vi "GeneratePadLookup.vi"(8 "error in (no error)":errorcluster, 11 "PadLookupRef":refnum<vi>) -> (0 "error out":errorcluster)   [LabVIEW 2012]
uses:
  Controls/PadLookup.ctl
  Controls/PadLookupItem.ctl
  Controls/PadArea.ctl
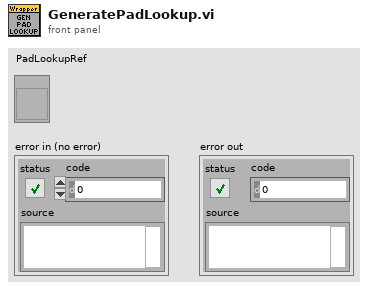
[diagram p1: front panel]
types:
  T1 = typedef "PadLookup.ctl" = cluster{"A":T2, "B":T2, "C":T2, "D":T2, "L":T2, "R":T2, "T":T2, "G":T2}
  T2 = typedef "PadLookupItem.ctl" = cluster{"PadArea":T3, string[]}
  T3 = typedef "PadArea.ctl" = enum16{"CenterA", "CenterB", "CenterC", "CenterD", "L", "R", "T", "G"}
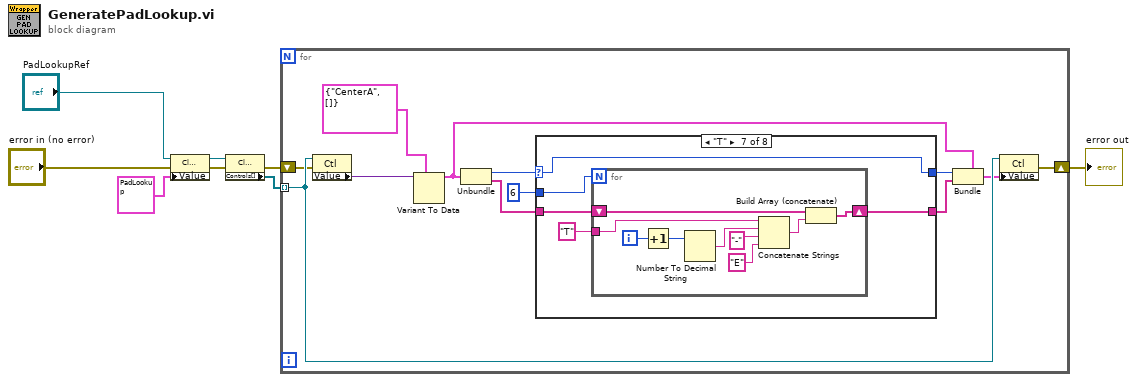
[diagram p0: block diagram]
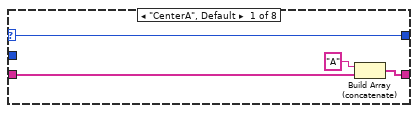
[diagram p2: hidden frame]
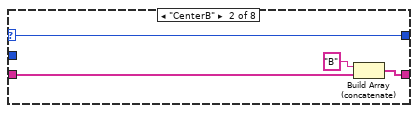
[diagram p3: hidden frame]
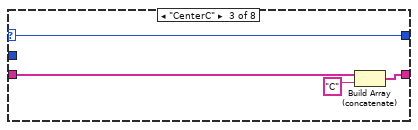
[diagram p4: hidden frame]
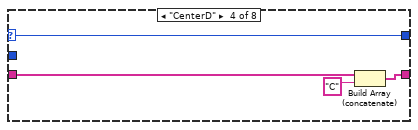
[diagram p5: hidden frame]
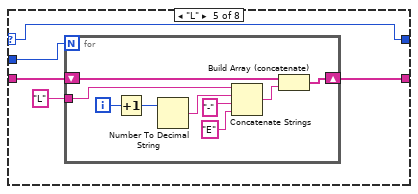
[diagram p6: hidden frame]
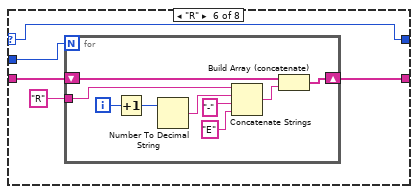
[diagram p7: hidden frame]
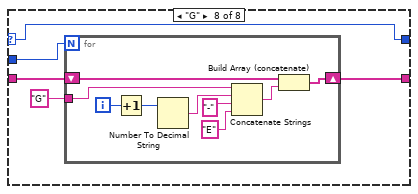
[diagram p8: hidden frame]
diagram:
  n1 = property class="Clust (strict)"(reference="PadLookupRef", error in="error in (no error)", "Value"=T1 {"A"={"PadArea"=enum."CenterA", []}, "B"={"PadArea"=enum."CenterB", []}, "C"={"PadArea"=enum."CenterC", []}, "D"={"PadArea"=enum."CenterD", []}, "L"={"PadArea"=enum."L", []}, "R"={"PadArea"=enum."R", []}, "T"={"PadArea"=enum."T", []}, "G"={"PadArea"=enum."G", []}} ("PadLookup")) -> (reference out=w4:refnum<vi>, error out=w5:errorcluster)
  n2 = property class="Clust (strict)"(reference=w4, error in=w5) -> (error out=w7:errorcluster, "Controls[]"=w3:refnum<vi>[])  [unwired: 1 out]
  n3 = for {
    tunnel: w3 -> [w15] mode=indexing
    shift-right: [w9] -> w8
    shift-left: w7 -> [w10]
    n4 = property class="Ctl"(reference=w15, error in=w10) -> ("Value"=w18:variant)  [unwired: 2 out]
    n5 = Variant To Data(type=T2 {"PadArea"=enum."CenterA", []} ("G"), Variant=w18) -> (data=w16:T2)  [unwired: 1 in, 1 out]
    n6 = Unbundle(w16) -> ("PadArea"=w12:T3, w20:string[])
    n7 = case shown="\"T\"" w12 {
      selector: w12 -> [w22 w26 w31 w34 w39 w53 w67 w81]
      tunnel: w20 -> [w24 w27 w32 w35 w41 w54 w68 w82]
      tunnel: [w22 w26 w31 w34 w39 w53 w67 w81] -> w19
      tunnel: [w21 w25 w29 w33 w40 w52 w66 w80] -> w13
      tunnel: 6 -> [_ _ _ _ w37 w51 w65 w79]
      frame "CenterA", Default {
        n8 = Build Array (concatenate)("A", w24) -> (w21:string[])
      }
      frame "CenterB" {
        n9 = Build Array (concatenate)("B", w27) -> (w25:string[])
      }
      frame "CenterC" {
        n10 = Build Array (concatenate)(w32, "C") -> (w29:string[])
      }
      frame "CenterD" {
        n11 = Build Array (concatenate)(w35, "C") -> (w33:string[])
      }
      frame "L" {
        n12 = for {
          N: w37 -> [_]
          shift-right: [w45] -> w40
          shift-left: w41 -> [w50]
          tunnel: "L" ("string") -> [w44]
          i -> [w49]
          n13 = Increment(x=w49) -> (x+1=w48:i32)
          n14 = Number To Decimal String(number=w48) -> (decimal integer string=w47:string)  [unwired: 1 in]
          n15 = Concatenate Strings(w44, w47, "-" ("string"), "E" ("string")) -> (w46:string)
          n16 = Build Array (concatenate)(w50, w46) -> (w45:string[])
        }
      }
      frame "R" {
        n17 = for {
          N: w51 -> [_]
          shift-right: [w59] -> w52
          shift-left: w54 -> [w64]
          tunnel: "R" ("string") -> [w58]
          i -> [w63]
          n18 = Increment(x=w63) -> (x+1=w62:i32)
          n19 = Number To Decimal String(number=w62) -> (decimal integer string=w61:string)  [unwired: 1 in]
          n20 = Concatenate Strings(w58, w61, "-" ("string"), "E" ("string")) -> (w60:string)
          n21 = Build Array (concatenate)(w64, w60) -> (w59:string[])
        }
      }
      frame "T" {
        n22 = for {
          N: w65 -> [_]
          shift-right: [w73] -> w66
          shift-left: w68 -> [w78]
          tunnel: "T" ("string") -> [w72]
          i -> [w77]
          n23 = Increment(x=w77) -> (x+1=w76:i32)
          n24 = Number To Decimal String(number=w76) -> (decimal integer string=w75:string)  [unwired: 1 in]
          n25 = Concatenate Strings(w72, w75, "-" ("string"), "E" ("string")) -> (w74:string)
          n26 = Build Array (concatenate)(w78, w74) -> (w73:string[])
        }
      }
      frame "G" {
        n27 = for {
          N: w79 -> [_]
          shift-right: [w87] -> w80
          shift-left: w82 -> [w92]
          tunnel: "G" ("string") -> [w86]
          i -> [w91]
          n28 = Increment(x=w91) -> (x+1=w90:i32)
          n29 = Number To Decimal String(number=w90) -> (decimal integer string=w89:string)  [unwired: 1 in]
          n30 = Concatenate Strings(w86, w89, "-" ("string"), "E" ("string")) -> (w88:string)
          n31 = Build Array (concatenate)(w92, w88) -> (w87:string[])
        }
      }
    }
    n32 = Bundle(cluster=w16, "PadArea"=w19, w13) -> (w14:T2)
    n33 = property class="Ctl"(reference=w15, "Value"=w14) -> (error out=w9:errorcluster)  [unwired: 1 in, 1 out]
  }
  "error out" <- w8
